vi "Get Answer and Reasoning.vi"(10 "openrouter reasoning":string, 11 "answer":string) -> (2 "reasoning":string, 3 "answer":string)   [LabVIEW 2023, in "LabVIEW LLM.lvlib"]
uses:
  LabVIEW LLM.lvlib
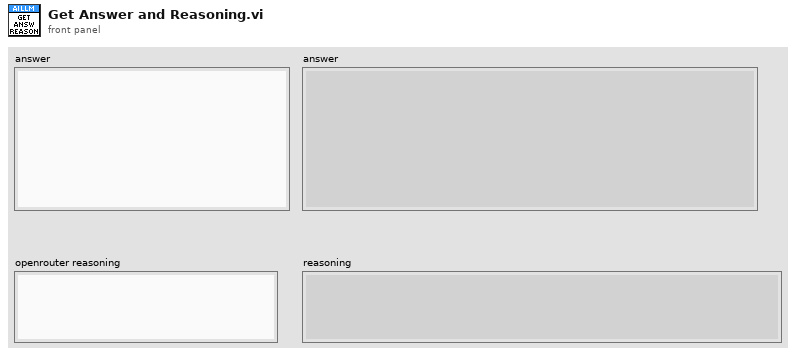
[diagram p1: front panel]
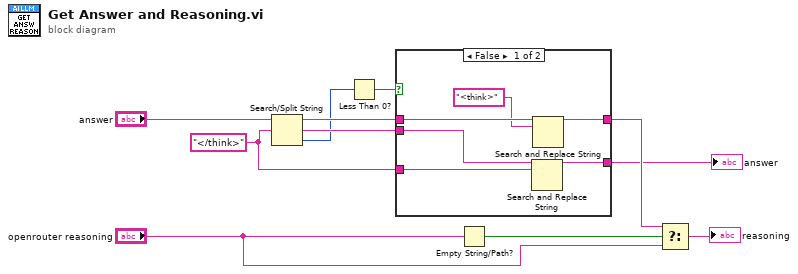
[diagram p0: block diagram]
diagram:
  w3 = "</think>" ("search string/char (-)")
  n1 = Search/Split String(string="answer", search string/char (-)=w3) -> (substring before match=w7:string, match + rest of string=w5:string, offset of match=w2:i32)  [unwired: 1 in]
  n2 = Less Than 0?(x=w2) -> (x < 0?=w1:bool)
  n3 = case shown="False" w1 {
    tunnel: w7 -> [w17 w18]
    tunnel: [w16 _] -> w6
    tunnel: w5 -> [w15 _]
    tunnel: [w14 w18] -> w4
    tunnel: w3 -> [w13 _]
    frame False {
      n4 = Search and Replace String(input string=w15, search string=w13) -> (result string=w14:string)  [unwired: 6 in, 3 out]
      n5 = Search and Replace String(input string=w17, search string="<think>" ("substring (\"\")")) -> (result string=w16:string)  [unwired: 6 in, 3 out]
    }
    frame True {
    }
  }
  "answer" <- w4
  n6 = Empty String/Path?(string/path="openrouter reasoning") -> (empty?=w10:bool)
  n7 = Select(t=w6, s=w10, f="openrouter reasoning") -> (s? t:f=→"reasoning":string)
